vi "Multitone with Amplitudes.vi"() -> ()   [LabVIEW 2023]
doc: "This VI demonstrates the use of the Basic Multitone with Amplitudes.vi. First, the desired amplitudes are generated. Then the multitone signal is created. Finally, the multitone signal is analyzed and displayed. Notice that the Basic Multitone with Amplitudes.vi may not generate all the requested tones due to Nyquist constraints. If some of the requested tones are not generated a warning is issued in the error out cluster."
uses:
  <vilib>/Analysis/4window.llb/windowTd.ctl
  <vilib>/Analysis/1siggen.llb/Ramp Pattern by Samples.vi
  <vilib>/measure/maspectr.llb/FFT Spectrum (Mag-Phase).vi
  <vilib>/measure/NI_MAPro.lvlib
  <vilib>/Analysis/NI_AALPro.lvlib
  <vilib>/Analysis/NI_AALBase.lvlib
panel:
  out "largest harmonic":dbl=39.0 format="%#.6g"
  out "# harmonics":i32=20
  out "Magnitude":cluster{"f0":dbl, "df":dbl, "magnitude":dbl[]}(graph)
  out "Time Waveform":waveform(dbl)(graph)
  # "Overview: Demonstrates the use of the Basic Multitone with Amplitudes VI.\nRequirements: LabVIEW Full Development System\nInstructions:\nRun the VI. Observe the original Time Waveform, and the Magnitude plot displaying the harmonics that result from performing an FFT on the signal."
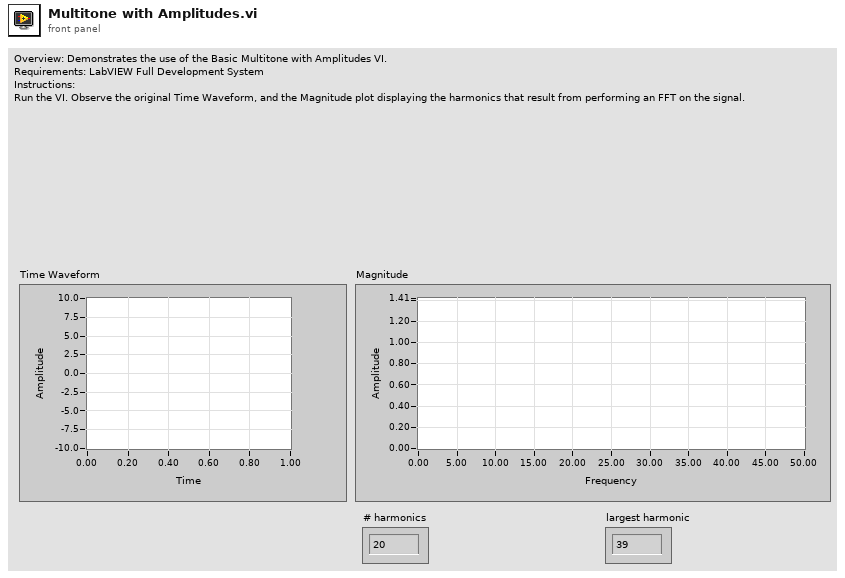
[diagram p1: front panel]
types:
  T1 = typedef "NI_AALPro.lvlib/windowTd.ctl" = u32
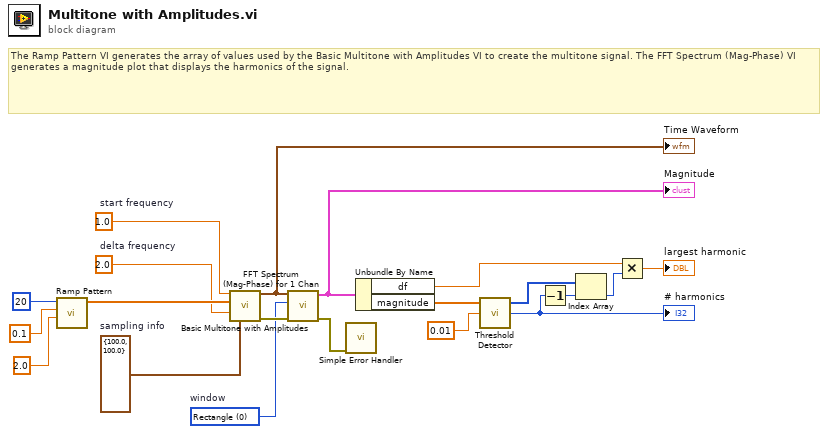
[diagram p0: block diagram]
diagram:
  w5 = T1 0 items=["Rectangle"=0, "Hanning"=1, "Hamming"=2, "Blackman-Harris"=3, "Exact Blackman"=4, "Blackman"=5, "Flat Top"=6, "4 Term B-Harris "=7, "7 Term B-Harris"=8, "Low Sidelobe"=9, "Blackman Nuttall"=11, "Triangle"=30, "Bartlett-Hanning"=31, "Bohman"=32, "Parzen"=33, "Welch"=34, "Kaiser"=60, "Dolph-Chebyshev"=61, "Gaussian"=62]  # window
  w17 = 2.0  # delta frequency
  w18 = cluster{"Fs":dbl, "#s":dbl} {"Fs"=100.0, "#s"=100.0}  # sampling info
  w16 = 1.0  # start frequency
  # "The Ramp Pattern VI generates the array of values used by the Basic Multitone with Amplitudes VI to create the multitone signal. The FFT Spectrum (Mag-Phase) VI generates a magnitude plot that displays the harmonics of the signal."
  n1 = call-poly <vilib>:"Ramp Pattern.vi"("start"=2.0, "end"=0.1, "samples"=20) -> ("Ramp Pattern"=w19:dbl[])  [unwired: 7 in, 1 out]
  n2 = call <vilib>:"Basic Multitone with Amplitudes.vi"("start frequency"=w16, "tone amplitudes"=w19, "delta frequency"=w17, "sampling info"=w18) -> ("signal out"=w15:waveform(dbl), "error out"=w13:errorcluster)  [unwired: 8 in, 2 out]
  "Time Waveform" <- w15
  n3 = call-poly <vilib>:"FFT Spectrum (Mag-Phase) for 1 Chan.vi"("error in (no error)"=w13, "window"=w5, "time signal"=w15) -> ("error out"=w20:errorcluster, "magnitude"=w12:cluster{"f0":dbl, "df":dbl, "magnitude":dbl[]})  [unwired: 4 in, 3 out]
  "Magnitude" <- w12
  n4 = call <vilib>:"Simple Error Handler.vi"("error in (no error)"=w20) -> ()  [unwired: 4 in, 5 out]
  n5 = Unbundle By Name(w12) -> ("df"=w6:dbl, "magnitude"=w11:dbl[])
  n6 = call <vilib>:"Threshold Detector.vi"("threshold"=0.01, "X"=w11) -> ("count"=w10:i32, "Indices"=w9:i32[])  [unwired: 1 in, 1 out]
  "# harmonics" <- w10
  n7 = Decrement(x=w10) -> (x-1=w14:i32)
  n8 = Index Array(array=w9, index=w14) -> (element=w8:i32)
  n9 = Multiply(x=w6, y=w8) -> (x*y=→"largest harmonic":dbl)
